vi "EasyVIAborter.vi"() -> ()   [LabVIEW 2013]
panel:
  in  "Filter Running?":bool=TRUE
  in  "Exit":bool
  in  "Abort!":bool
  in  "Select VI to abort":i32[](listbox)
  # "Easy VI Aborter"
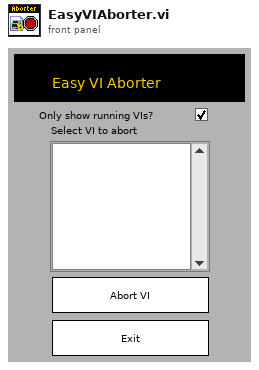
[diagram p1: front panel]
types:
  T1 = enum32{"Bad", "Idle", "Run top level", "Running"}
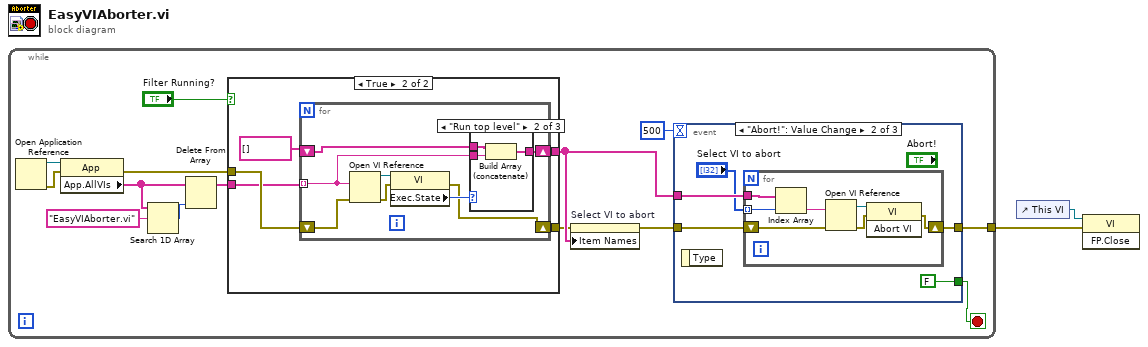
[diagram p0: block diagram]
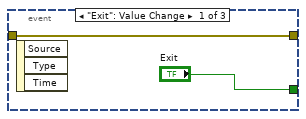
[diagram p2: hidden frame]
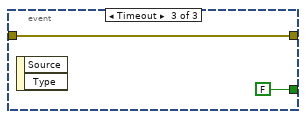
[diagram p3: hidden frame]
diagram:
  n1 = while {
    tunnel: [w13] -> w1
    stop <- w4 stop-if-true
    n2 = Open Application Reference() -> (0:w15:errorcluster, 3:w16:refnum<vi>)  [unwired: 1 in, 3 out]
    n3 = property class="App"(reference=w16, error in=w15) -> (error out=w10:errorcluster, "App.AllVIs"=w8:string[])  [unwired: 1 out]
    n4 = Search 1D Array(1D array=w8, element="EasyVIAborter.vi") -> (index of element=w7:i32)  [unwired: 1 out]
    n5 = Delete From Array(array=w8, index=w7) -> (array with subset deleted=w6:string[])  [unwired: 1 in, 1 out]
    n6 = case shown="True" "Filter Running?" {
      tunnel: [w34 w39] -> w12
      tunnel: [w33 w38] -> w11
      tunnel: w10 -> [w33 w37]
      tunnel: w6 -> [w34 w35]
      frame False {
      }
      frame True {
        n7 = for {
          tunnel: w35 -> [w45] mode=indexing
          shift-right: [w44] -> w39
          shift-left: string[] [] -> [w43]
          shift-right: [w41] -> w38
          shift-left: w37 -> [w40]
          n8 = Open VI Reference(vi path=w45, error in (no error)=w40) -> (vi reference=w47:refnum<vi>, error out=w42:errorcluster)  [unwired: 4 out]
          n9 = property class="VI"(reference=w47, error in=w42) -> (error out=w41:errorcluster, "Exec.State"=w46:T1)  [unwired: 1 out]
          n10 = case shown="\"Run top level\"" w46 {
            tunnel: w45 -> [_ w50 _]
            tunnel: [w48 w49 w52] -> w44
            tunnel: w43 -> [w48 w51 w52]
            frame "Bad", "Idle", Default {
            }
            frame "Run top level" {
              n11 = Build Array (concatenate)(w51, w50) -> (w49:string[])
            }
            frame "Running" {
            }
          }
        }
      }
    }
    n12 = property on="Select VI to abort" class="LstBox (strict)"(error in=w11, "Item Names"=w12) -> (error out=w14:errorcluster)  [unwired: 1 in, 1 out]
    n13 = event shown="[1] \"Abort!\": Value Change" {
      selector: _ -> [_ _ _]
      dyn-events: _ -> [_ _ _]
      timeout: 500 -> [_ _ _]
      tunnel: w12 -> [_ w23 _]
      tunnel: w14 -> [w18 w21 w32]
      tunnel: [w18 w20 w32] -> w13
      tunnel: ["Exit" FALSE ("Exit") FALSE ("Exit")] -> w4
      event "Exit": Value Change {
        n14 = event-data() -> ()  [unwired: 4 out]
      }
      event "Abort!": Value Change {
        n15 = event-data() -> ()  [unwired: 2 out]
        n16 = for {
          tunnel: w23 -> [w29]
          tunnel: "Select VI to abort" -> [w28] mode=indexing
          shift-right: [w24] -> w20
          shift-left: w21 -> [w26]
          n17 = Index Array(array=w29, index=w28) -> (element=w27:string)
          n18 = Open VI Reference(vi path=w27, error in (no error)=w26) -> (vi reference=w30:refnum<vi>, error out=w25:errorcluster)  [unwired: 4 out]
          n19 = invoke class="VI" method="Abort VI"(reference=w30, error in=w25) -> (error out=w24:errorcluster)  [unwired: 1 in, 2 out]
        }
      }
      event Timeout {
        n20 = event-data() -> ()  [unwired: 3 out]
      }
    }
  }
  n21 = control-ref of="This VI"() -> (w2:refnum<vi>)
  n22 = invoke class="VI" method="FP.Close"(reference=w2, error in=w1) -> ()  [unwired: 1 in, 3 out]
